vi "TEST Get VI Event Structure Reference.vi"(8 "error in (no error)":errorcluster) -> (0 "error out":errorcluster)   [LabVIEW 2020, in "TEST JKI State Machine API.lvlib"]
uses:
  TEST JKI State Machine API.lvlib
  <vilib>/addons/_JKI Toolkits/Caraya/classes/Test/Test.lvclass
  source/JKI SM/JKI SM.lvclass
  <vilib>/addons/_JKI Toolkits/Caraya/classes/Assert/Assert.lvclass
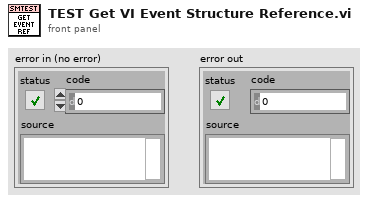
[diagram p1: front panel]
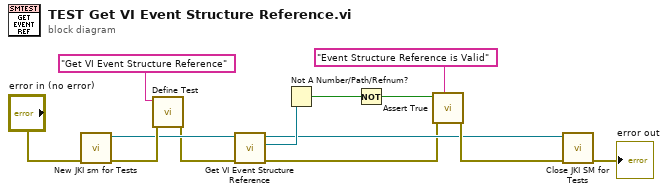
[diagram p0: block diagram]
diagram:
  n1 = call "New JKI sm for Tests.vi"("error in (no error)"="error in (no error)") -> ("error out"=w13:errorcluster, "JKI SM out"=w7:refnum<class "JKI SM.lvclass">)  [unwired: 9 in]
  n2 = call <vilib>:"Define Test.vi"("error in (no error)"=w13, "Label (VI Title)"="Get VI Event Structure Reference") -> ("error out"=w6:errorcluster)  [unwired: 8 in, 1 out]
  n3 = call "Get VI Event Structure Reference.vi"("error in (no error)"=w6, "JKI SM in"=w7) -> ("error out"=w2:errorcluster, "Event Structure ref"=w5:refnum<vi>, "JKI SM out"=w3:refnum<class "JKI SM.lvclass">)  [unwired: 7 in]
  n4 = Not A Number/Path/Refnum?(number/path/refnum=w5) -> (NaN/Path/Refnum?=w4:bool)
  n5 = Not(x=w4) -> (.not. x?=w1:bool)
  n6 = call <vilib>:"Assert True.vi"("Label"="Event Structure Reference is Valid", "error in (no error)"=w2, "True?"=w1) -> ("error out"=w10:errorcluster)  [unwired: 7 in, 1 out]
  n7 = call "Close JKI SM for Tests.vi"("error in (no error)"=w10, "JKI SM in"=w3) -> ("error out"=→"error out":errorcluster)  [unwired: 9 in]
